vi "VoltageCurrent.vi"() -> ()   [LabVIEW 2017]
uses:
  <vilib>/Instr/_visa.llb/VISA Configure Serial Port (Instr).vi
  <vilib>/Analysis/NI_AALPro.lvlib
panel:
  out "Voltage, V":string[][](table)
  out "Bytes at Port":u32
  out "Current, mA":string[][](table)
  out "V-I characteristic":cluster{"Y":dbl[], "Y":dbl[]}[](graph) caption="XY Graph"
  out "current":dbl format="%.2f"
  out "voltage":dbl format="%.2f"
  in  "baud rate (9600)":u32=9600
  in  "VISA resource name":refnum<visa-resource-name>
  in  "Stop":bool
  out "read buffer":string
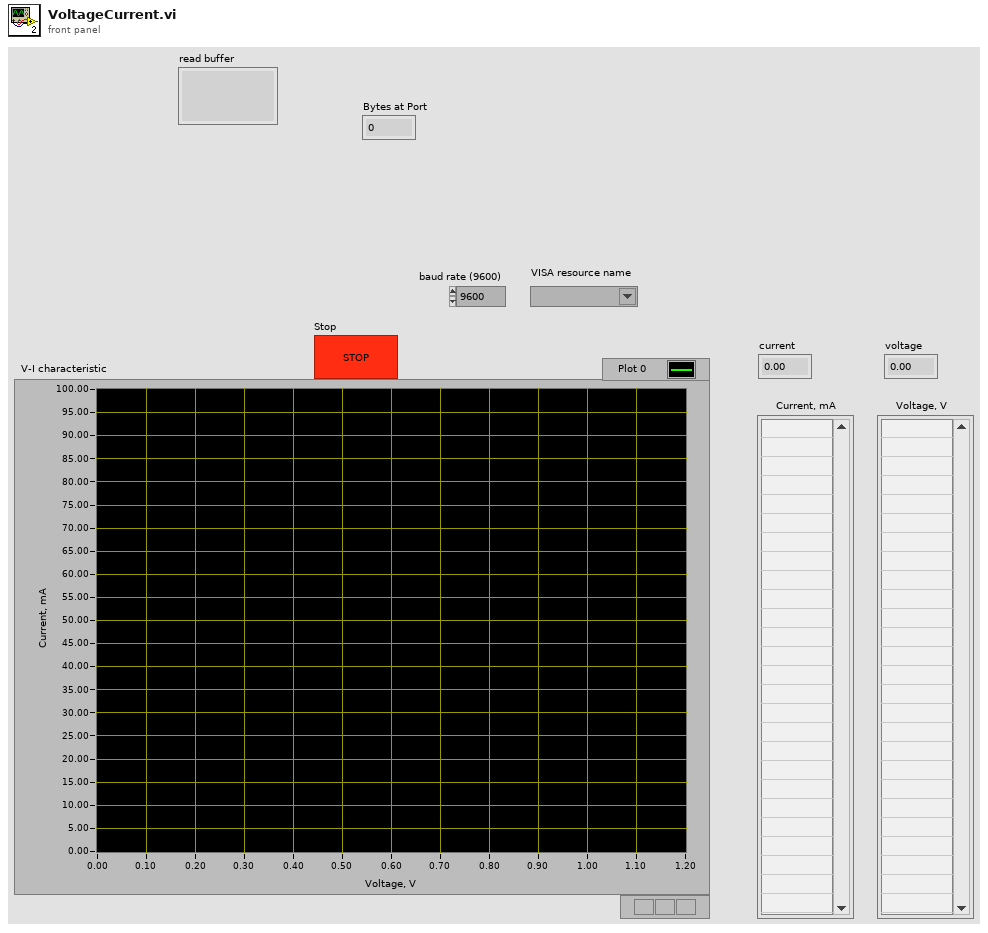
[diagram p1: front panel]
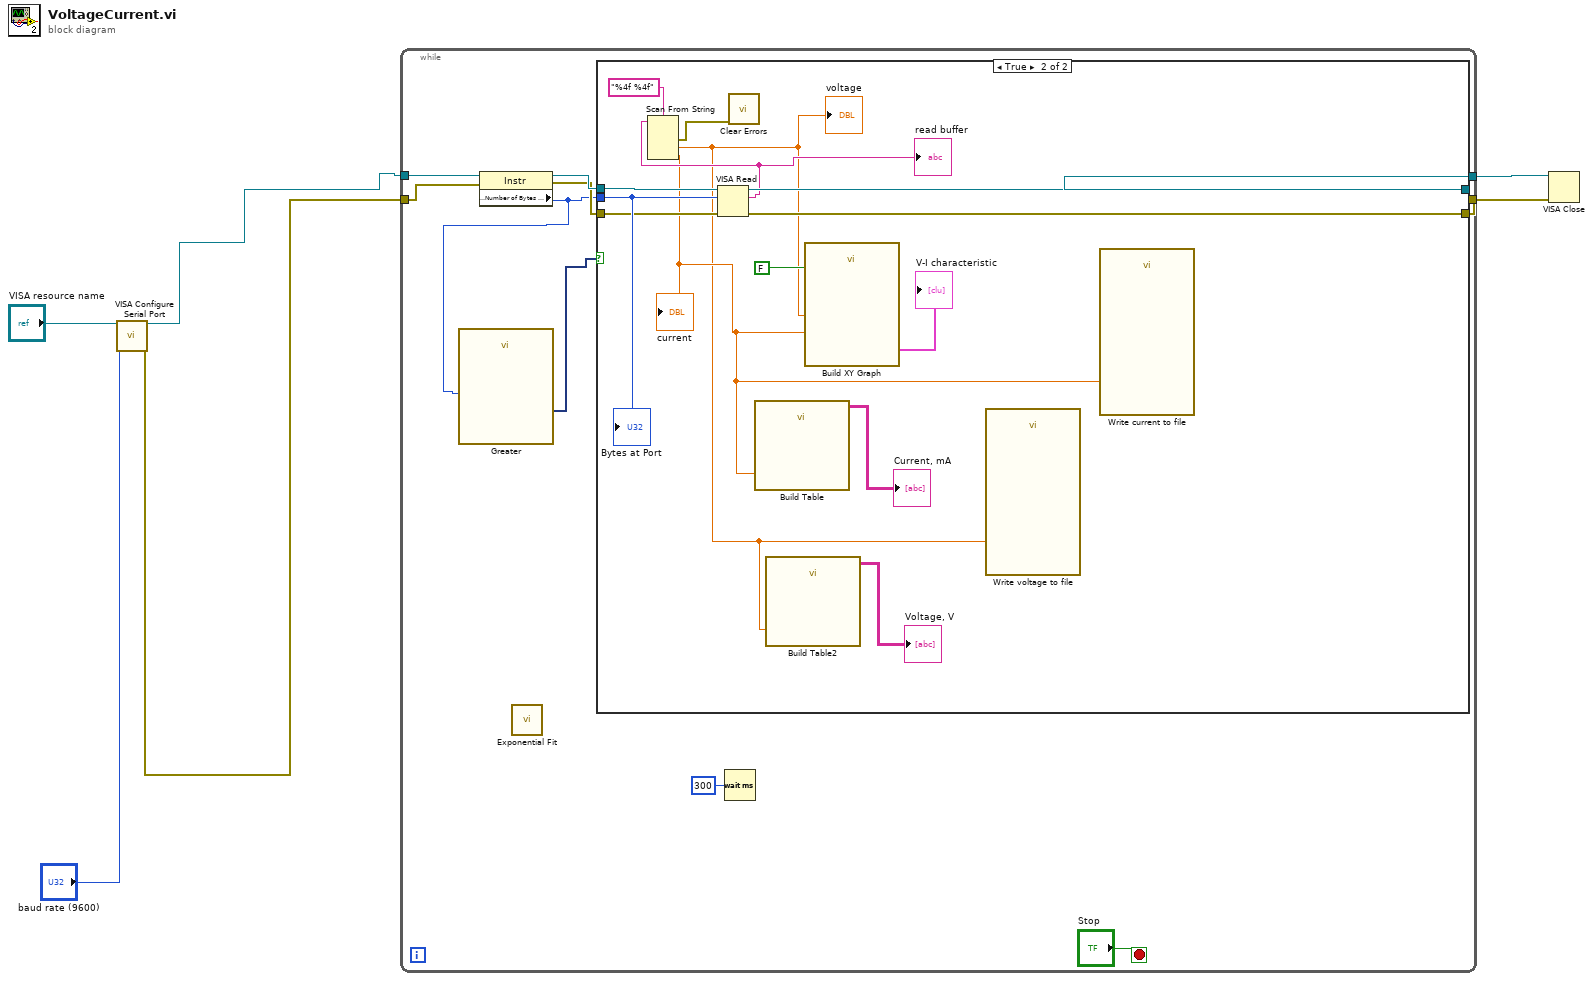
[diagram p0: block diagram]
diagram:
  n1 = call-poly "VISA Configure Serial Port"("VISA resource name"="VISA resource name", "baud rate (9600)"="baud rate (9600)") -> ("VISA resource name out"=w2:refnum<visa-resource-name>, "error out"=w1:errorcluster)  [unwired: 12 in]
  n2 = while {
    tunnel: w2 -> [w15]
    tunnel: w1 -> [w14]
    tunnel: [w11] -> w6
    tunnel: [w10] -> w5
    stop <- "Stop" stop-if-true
    n3 = property class="Instr"(reference=w15, error in=w14) -> (reference out=w13:refnum<visa-resource-name>, error out=w12:errorcluster, "Serial Settings:Number of Bytes at Serial Port"=w8:u32)
    n4 = call "Greater"("Operand 1"=w8) -> ("Result"=w7:dynamicdata)  [unwired: 9 in, 1 out]
    n5 = call <vilib>:"Exponential Fit.vi"() -> ()  [unwired: 10 in, 6 out]
    n6 = case shown="True" w7 {
      tunnel: w8 -> [_ w32]
      tunnel: w13 -> [w18 w31]
      tunnel: w12 -> [w17 w30]
      tunnel: [w17 w29] -> w11
      tunnel: [w18 w28] -> w10
      frame False {
      }
      frame True {
        n7 = VISA Read(VISA resource name=w31, byte count=w32, error in (no error)=w30) -> (VISA resource name out=w28:refnum<visa-resource-name>, read buffer=w27:string, error out=w29:errorcluster)  [unwired: 1 out]
        "read buffer" <- w27
        n8 = Scan From String(format string="%4f %4f", input string=w27) -> (error out=w21:errorcluster, output 1=w19:dbl, output 2=w22:dbl)  [unwired: 4 in, 2 out]
        "voltage" <- w19
        "current" <- w22
        n9 = call <vilib>:"Clear Errors.vi"("error in (no error)"=w21) -> ()  [unwired: 5 in, 2 out]
        n10 = call "Build Table"("Signals"=w22) -> ("Table"=→"Current, mA":string[][])  [unwired: 4 in, 6 out]
        n11 = call "Build Table2"("Signals"=w19) -> ("Table"=→"Voltage, V":string[][])  [unwired: 4 in, 6 out]
        n12 = call "Build XY Graph"("Reset"=FALSE, "Y Input"=w22, "X Input"=w19) -> ("XY Graph"=→"V-I characteristic":cluster{"X":dbl[], "Y":dbl[]}[])  [unwired: 7 in, 1 out]
        n13 = call "Write voltage to file"("Signals"=w19) -> ()  [unwired: 16 in, 3 out]
        n14 = call "Write current to file"("Signals"=w22) -> ()  [unwired: 16 in, 3 out]
        "Bytes at Port" <- w32
      }
    }
    n15 = Wait (ms)(milliseconds to wait=u32 300) -> ()  [unwired: 1 out]
  }
  n16 = VISA Close(VISA resource name=w5, error in (no error)=w6) -> ()  [unwired: 1 out]
